vi "TCP Scanner.vi"(3 "Port（4001）":u16=4001, 4 "超时毫秒(100)":i32=500, 5 "byte of read(9)":i32=9, 6 "ip":string) -> (0 "status":bool, 1 "错误输出":errorcluster, 2 "Barcode":string)   [LabVIEW 2018]
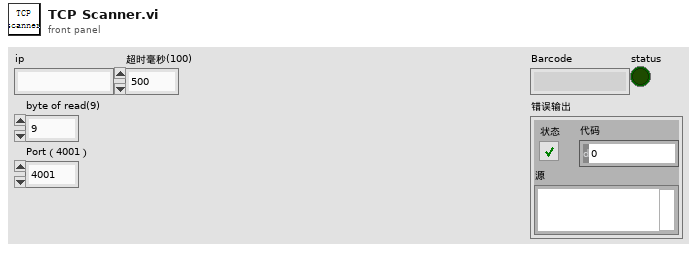
[diagram p1: front panel]
types:
  T1 = enum16{"Standard", "Buffered", "CRLF", "Immediate"}
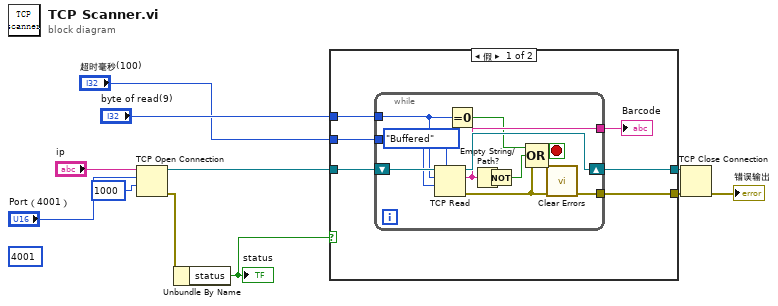
[diagram p0: block diagram]
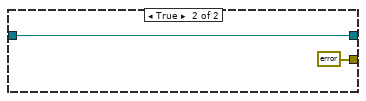
[diagram p2: hidden frame]
diagram:
  (unwired) u16 4001 ("远程端口或服务名称")
  n1 = TCP Open Connection(address="ip", remote port or service name="Port（4001）", timeout ms (60000)=1000 ("超时毫秒(60000)")) -> (connection ID=w10:refnum<k5>, error out=w3:errorcluster)  [unwired: 2 in]
  n2 = Unbundle By Name(w3) -> ("status"=w2:bool)
  "status" <- w2
  n3 = case shown="假" w2 {
    tunnel: w10 -> [w16 w31]
    tunnel: [w15 w31] -> w9
    tunnel: [w14 errorcluster {"status"=FALSE, "code"=0, "source"=""} ("error out")] -> w8
    tunnel: "超时毫秒(100)" -> [w13 _]
    tunnel: "byte of read(9)" -> [w12 _]
    frame False {
      n4 = while {
        tunnel: [w25] -> w17
        tunnel: w13 -> [w27]
        tunnel: w12 -> [w23]
        shift-right: [w28] -> w15
        shift-left: w16 -> [w29]
        tunnel: [w26] -> w14
        stop <- w20 stop-if-true
        n5 = TCP Read(connection ID=w29, bytes to read=w23, 7:T1."Buffered" ("模式（标准）"), 9:w27) -> (connection ID out=w28:refnum<k5>, data out=w25:string, error out=w19:errorcluster)  [unwired: 1 in]
        n6 = Equal To 0?(x=w23) -> (x = 0?=w21:bool)
        n7 = Empty String/Path?(string/path=w25) -> (empty?=w24:bool)
        n8 = Not(x=w24) -> (.not. x?=w22:bool)
        n9 = Compound Arithmetic op=OR ("复合运算")(w21, w22, w19) -> (w20:bool)
        n10 = call <vilib>:"Clear Errors.vi"("error in (no error)"=w19) -> ("error out"=w26:errorcluster)  [unwired: 5 in, 1 out]
      }
      "Barcode" <- w17
    }
    frame True {
    }
  }
  n11 = TCP Close Connection(connection ID=w9, error in (no error)=w8) -> (error out=→"错误输出":errorcluster)  [unwired: 1 in, 1 out]
